vi "delete later.vi"() -> ()   [LabVIEW 2021]
uses:
  controls/TCP states.ctl
  9f39ed20-5445-4280-9795-060522750320.vi
  6f00eeef-efb4-482c-a3e2-20a697cd7ee2.vi
  28ccb5b7-2f25-45df-bbde-98550ad008d4.vi
  c062eeae-77f3-4d9f-bdcd-b3742af7fc49.vi
panel:
  out "Response 3":string
  out "Response 2":string
  out "Response":string
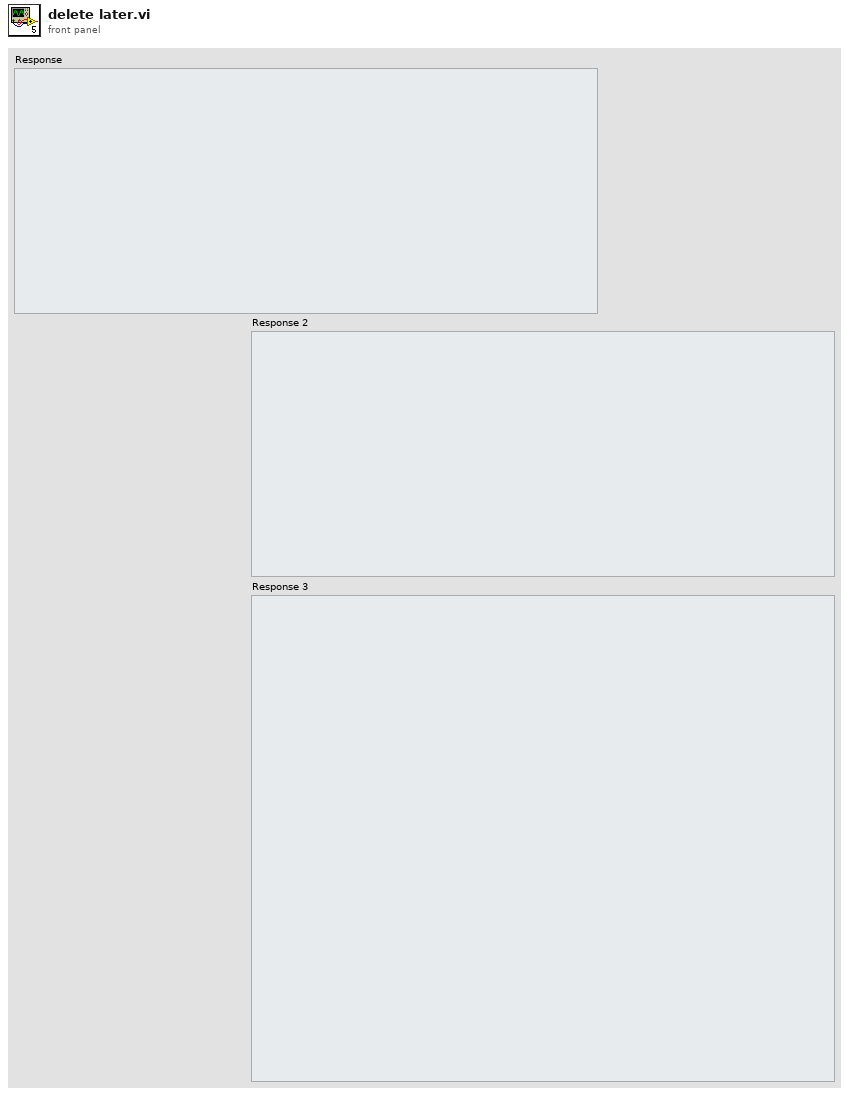
[diagram p1: front panel]
types:
  T1 = typedef "TCP states.ctl" = string
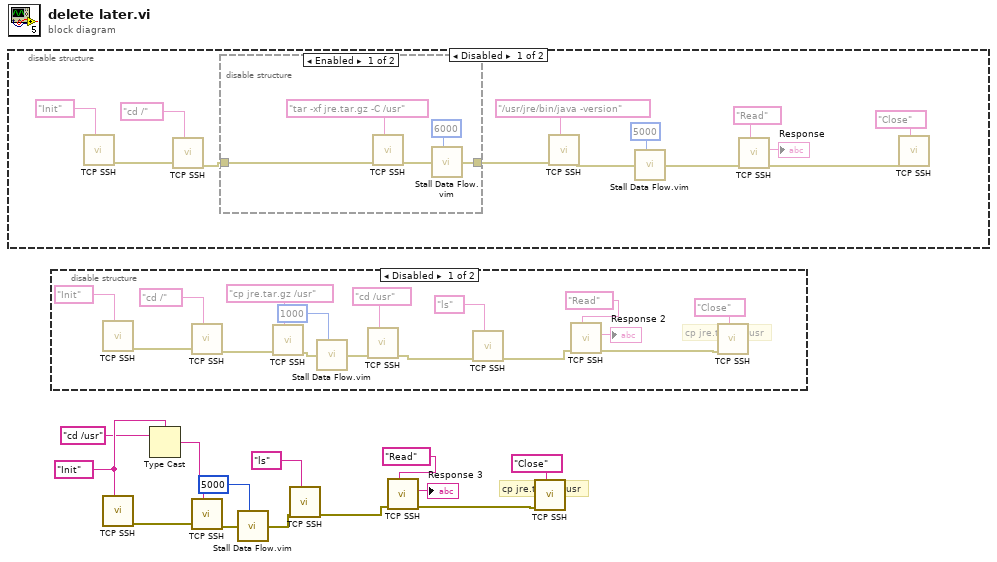
[diagram p0: block diagram]
diagram:
  w5 = T1 "Init" ("States")
  # "cp jre.tar.gz /usr"
  n1 = disable-structure shown="Disabled" {
    frame Disabled {
      n2 = call "TCP SSH.vi"("States"=T1 "Init") -> ("Error  Out"=w15:errorcluster)  [unwired: 8 in, 1 out]
      n3 = call "TCP SSH.vi"("States"=T1 "cd /", "Error In"=w15) -> ("Error  Out"=w14:errorcluster)  [unwired: 7 in, 1 out]
      n4 = disable-structure shown="Enabled" {
        disable-tunnel: w14 -> [w31 w32]
        disable-tunnel: [w28 w32] -> w24
        frame Enabled {
          n5 = call "TCP SSH.vi"("States"=T1 "tar -xf jre.tar.gz -C /usr", "Error In"=w31) -> ("Error  Out"=w30:errorcluster)  [unwired: 7 in, 1 out]
          n6 = call "Stall Data Flow.vim"("value in"=w30, "milliseconds to wait"=u32 6000) -> ("value out"=w28:errorcluster)  [unwired: 1 out]
        }
        frame Disabled {
        }
      }
      n7 = call "TCP SSH.vi"("States"=T1 "/usr/jre/bin/java -version", "Error In"=w24) -> ("Error  Out"=w22:errorcluster)  [unwired: 7 in, 1 out]
      n8 = call "Stall Data Flow.vim"("value in"=w22, "milliseconds to wait"=u32 5000) -> ("value out"=w18:errorcluster)  [unwired: 1 out]
      n9 = call "TCP SSH.vi"("States"=T1 "Read", "Error In"=w18) -> ("Error  Out"=w21:errorcluster, "Response"=→"Response":string)  [unwired: 7 in]
      n10 = call "TCP SSH.vi"("States"=T1 "Close", "Error In"=w21) -> ()  [unwired: 7 in, 2 out]
    }
    frame Enabled {
    }
  }
  n11 = disable-structure shown="Disabled" {
    frame Disabled {
      # "cp jre.tar.gz /usr"
      n12 = call "TCP SSH.vi"("States"=T1 "Init") -> ("Error  Out"=w46:errorcluster)  [unwired: 8 in, 1 out]
      n13 = call "TCP SSH.vi"("States"=T1 "cd /", "Error In"=w46) -> ("Error  Out"=w44:errorcluster)  [unwired: 7 in, 1 out]
      n14 = call "TCP SSH.vi"("States"=T1 "cp jre.tar.gz /usr", "Error In"=w44) -> ("Error  Out"=w38:errorcluster)  [unwired: 7 in, 1 out]
      n15 = call "Stall Data Flow.vim"("value in"=w38, "milliseconds to wait"=u32 1000) -> ("value out"=w34:errorcluster)  [unwired: 1 out]
      n16 = call "TCP SSH.vi"("States"=T1 "cd /usr", "Error In"=w34) -> ("Error  Out"=w36:errorcluster)  [unwired: 7 in, 1 out]
      n17 = call "TCP SSH.vi"("States"=T1 "ls", "Error In"=w36) -> ("Error  Out"=w35:errorcluster)  [unwired: 7 in, 1 out]
      n18 = call "TCP SSH.vi"("States"=T1 "Read", "Error In"=w35) -> ("Error  Out"=w40:errorcluster, "Response"=→"Response 2":string)  [unwired: 7 in]
      n19 = call "TCP SSH.vi"("States"=T1 "Close", "Error In"=w40) -> ()  [unwired: 7 in, 2 out]
    }
    frame Enabled {
    }
  }
  n20 = call "TCP SSH.vi"("States"=w5) -> ("Error  Out"=w13:errorcluster)  [unwired: 8 in, 1 out]
  n21 = Type Cast(type=w5, x="cd /usr") -> (*(type *) &x=w3:T1)
  n22 = call "TCP SSH.vi"("States"=w3, "Error In"=w13) -> ("Error  Out"=w7:errorcluster)  [unwired: 7 in, 1 out]
  n23 = call "Stall Data Flow.vim"("value in"=w7, "milliseconds to wait"=u32 5000) -> ("value out"=w2:errorcluster)  [unwired: 1 out]
  n24 = call "TCP SSH.vi"("States"=T1 "ls", "Error In"=w2) -> ("Error  Out"=w8:errorcluster)  [unwired: 7 in, 1 out]
  n25 = call "TCP SSH.vi"("States"=T1 "Read", "Error In"=w8) -> ("Error  Out"=w9:errorcluster, "Response"=→"Response 3":string)  [unwired: 7 in]
  n26 = call "TCP SSH.vi"("States"=T1 "Close", "Error In"=w9) -> ()  [unwired: 7 in, 2 out]
